vi "StateSpaceObserver.vi"(6 "Reinitialize":bool, 8 "X_hat_Initial":T1, 9 "u":dbl, 10 "y":dbl, 11 "Gains":T2) -> (3 "X_hat":T1)   [LabVIEW 2017]
uses:
  <vilib>/Analysis/Matrix/Datatypes/RealMatrix.ctl
  <vilib>/Analysis/baseanly.llb/Real A x B.vi
  <vilib>/Analysis/Matrix/Numeric/Multiply/Multiply - RM,R.vi
  <vilib>/Analysis/Matrix/Numeric/Add/Add - RM,RM.vi
  <vilib>/Analysis/NI_AALBase.lvlib
  <vilib>/Analysis/Matrix/NI_Matrix.lvlib
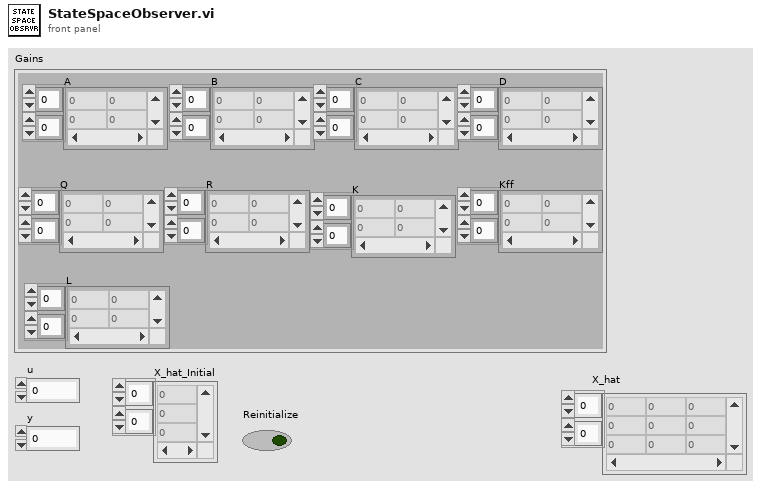
[diagram p1: front panel]
types:
  T1 = typedef "NI_Matrix.lvlib/RealMatrix.ctl" = dbl[][]
  T2 = cluster{"A":T1, "B":T1, "C":T1, "D":T1, "Q":T1, "R":T1, "K":T1, "Kff":T1, "L":T1}
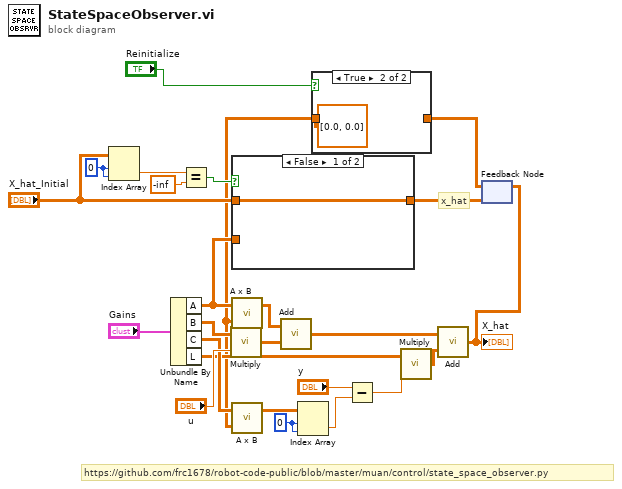
[diagram p0: block diagram]
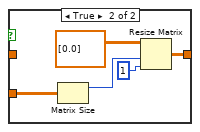
[diagram p3: hidden frame]
diagram:
  w10 = 0 ("index (row)")
  w16 = 0 ("index (row)")
  # "https://github.com/frc1678/robot-code-public/blob/master/muan/control/state_space_observer.py"
  # "x_hat"
  n1 = Index Array(array="X_hat_Initial", index (row)=w10, index (col)=w10) -> (element=w9:dbl)
  n2 = Unbundle By Name("Gains") -> ("A"=w7:T1, "B"=w24:T1, "C"=w18:T1, "L"=w14:T1)
  n3 = Equal?(x=w9, y=-inf) -> (x = y?=w5:bool)
  n4 = call-poly <vilib>:"Multiply.vi"("Real Scalar c"="u", "Real Matrix A"=w24) -> ("A * c"=w21:T1)
  n5 = case shown="False" w5 {
    tunnel: w7 -> [_ w28]
    tunnel: [w26 w27] -> w6
    tunnel: "X_hat_Initial" -> [w26 _]
    frame False {
    }
    frame True {
      n6 = Matrix Size(0:w28) -> (1:w31:i32)  [unwired: 1 out]
      n7 = Resize Matrix(1:1 ("number of columns"), 2:w31, 4:T1 [[0.0]] ("matrix")) -> (0:w27:T1)
    }
  }
  n8 = feedback #1(w6) -> (w2:T1)
  n9 = case shown="True" "Reinitialize" {
    tunnel: w2 -> [w32 _]
    tunnel: [w32 T1 [[0.0], [0.0]] ("matrix")] -> w1
    frame False {
    }
    frame True {
    }
  }
  n10 = call-poly <vilib>:"A x B.vi"("B"=w1, "A"=w7) -> ("A x B"=w22:T1)  [unwired: 1 out]
  n11 = call-poly <vilib>:"A x B.vi"("B"=w1, "A"=w18) -> ("A x B"=w17:T1)  [unwired: 1 out]
  n12 = call-poly <vilib>:"Add.vi"("Real Matrix B"=w21, "Real Matrix A"=w22) -> ("A + B"=w20:T1)
  n13 = Index Array(array=w17, index (row)=w16, index (col)=w16) -> (element=w15:dbl)
  n14 = Subtract(x="y", y=w15) -> (x-y=w13:dbl)
  n15 = call-poly <vilib>:"Multiply.vi"("Real Scalar c"=w13, "Real Matrix A"=w14) -> ("A * c"=w12:T1)
  n16 = call-poly <vilib>:"Add.vi"("Real Matrix B"=w12, "Real Matrix A"=w20) -> ("A + B"=w11:T1)
  "X_hat" <- w11
  n17 = feedback-in #1(w11) -> ()
